vi "FTW-Messenger-AsynchronousInit.vi"(0 "Messenger":refnum<class "FTW-Messenger.lvclass">, 5 "Initialized Response":refnum<class "FTW-Container.lvclass">, 11 "error in":errorcluster) -> (4 "Initialized Messenger":refnum<class "FTW-Messenger.lvclass">, 6 "Observer":refnum<event-registration>, 15 "error out":errorcluster)   [LabVIEW 2015, in "FTW-Messenger.lvclass"]
uses:
  FTW-Messenger.lvclass
  Message/FTW-Message.lvclass
  Container/FTW-Container.lvclass
  FTW-Messenger.lvclass/FTW-Messenger.ctl
panel:
  # "Inputs"
  # "Outputs"
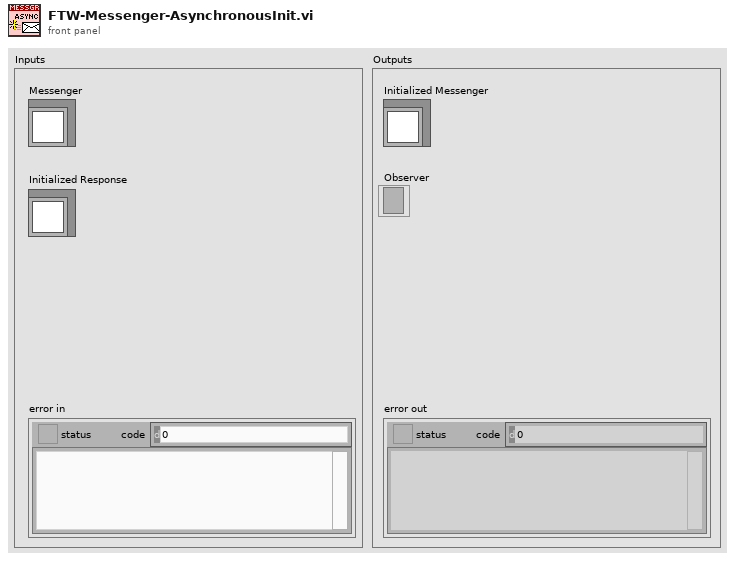
[diagram p1: front panel]
types:
  T1 = cluster{"Initialized Response":refnum<class "FTW-Container.lvclass">, "Messenger out":refnum<class "FTW-Messenger.lvclass">}
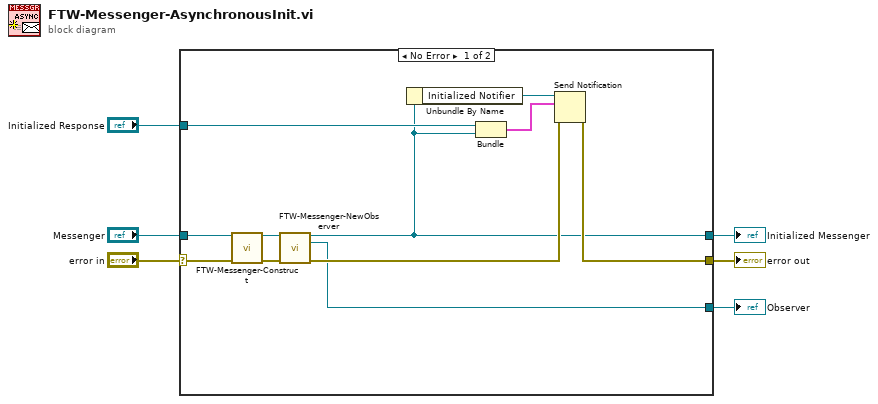
[diagram p0: block diagram]
diagram:
  n1 = case shown="No Error" "error in" {
    selector: "error in" -> [w11 w19]
    tunnel: [w17 w19] -> w4
    tunnel: [w7 w18] -> w5
    tunnel: "Messenger" -> [w9 w18]
    tunnel: "Initialized Response" -> [w10 _]
    tunnel: [w14 _] -> w2
    frame No Error {
      n2 = call-dynamic "FTW-Messenger-Construct.vi"("Messenger Type"=w9, "error in"=w11) -> ("Messenger"=w13:refnum<class "FTW-Messenger.lvclass">, "error out"=w16:errorcluster)  [unwired: 12 in]
      n3 = call "FTW-Messenger-NewObserver.vi"("Messenger"=w13, "error in"=w16) -> ("Messenger out"=w7:refnum<class "FTW-Messenger.lvclass">, "Message"=w14:refnum<event-registration>, "error out"=w15:errorcluster)  [unwired: 11 in]
      n4 = Unbundle By Name(w7) -> ("Initialized Notifier"=w8:refnum<notifier>)
      n5 = Bundle("Initialized Response"=w10, "Messenger out"=w7) -> (w12:T1)  [unwired: 1 in]
      n6 = Send Notification(notification=w12, notifier=w8, error in (no error)=w15) -> (error out=w17:errorcluster)  [unwired: 1 out]
    }
    frame Error {
    }
  }
  "Initialized Messenger" <- w5
  "error out" <- w4
  "Observer" <- w2
